vi "Create Input Channels.vi"(8 "error in (no error)":errorcluster, 11 "DAQmx Digitizer in":refnum<class "DAQmx Digitizer.lvclass">) -> (0 "error out":errorcluster, 3 "DAQmx Digitizer out":refnum<class "DAQmx Digitizer.lvclass">)   [LabVIEW 2024, in "DAQmx Digitizer.lvclass"]
uses:
  DAQmx Digitizer.lvclass
  DAQmx Digitizer.lvclass/DAQmx Digitizer.ctl
  Instruments/Pulse Driver/Pulse Driver.lvclass/Pulse Driver.ctl
  Instruments/Instrument Driver/Instrument Driver.lvclass/Instrument Driver.ctl
  Instruments/Pulse Driver/Read Pretrigger samples.vi
  Instruments/Pulse Driver/Read Samples per channel.vi
  Instruments/Instrument Driver/Read Type ID.vi
  Instruments/Pulse Driver/Write t0.vi
  Instruments/Pulse Driver/Write dt.vi
  Instruments/Pulse Driver/Write Set timing from UI.vi
  <vilib>/DAQmx/create/channels.llb/DAQmx Create Channel (AI-Voltage-Basic).vi
  <vilib>/DAQmx/configure/timing.llb/DAQmx Timing (Sample Clock).vi
  <vilib>/DAQmx/configure/trigger.llb/DAQmx Reference Trigger (Digital Edge).vi
  <vilib>/Utility/error.llb/Error Cluster From Error Code.vi
  <vilib>/DAQmx/configure/trigger.llb/DAQmx Start Trigger (Digital Edge).vi
  <vilib>/DAQmx/configure/events/hardwareSignals.llb/DAQmx Export Signal (Most Signals).vi
  <vilib>/ErrorRing/Error Ring.xnode
  <resource>/objmgr/daqmx.rc
  File/File Class/File.lvclass
panel:
  out "CompactDAQ.ChassisDevName":tag
  out "ProductCategory":i32(ring)=14643 items=["M Series DAQ"=14643, "X Series DAQ"=15858, "E Series DAQ"=14642, "S Series DAQ"=14644, "B Series DAQ"=14662, "SC Series DAQ"=14645, "USB DAQ"=14646, "AO Series"=14647, "Digital I/O"=14648, "TIO Series"=14661, "Dynamic Signal Acquisition"=14649, "Switches"=14650, "CompactDAQ Chassis"=14658, "CompactRIO Chassis"=16144, "C Series Module"=14659, "SCXI Module"=14660, "SCC Connector Block"=14704, "SCC Module"=14705, "NI ELVIS"=14755, "Network DAQ"=14829, "SC Express"=15886, "FieldDAQ"=16151, "Unknown"=12588]
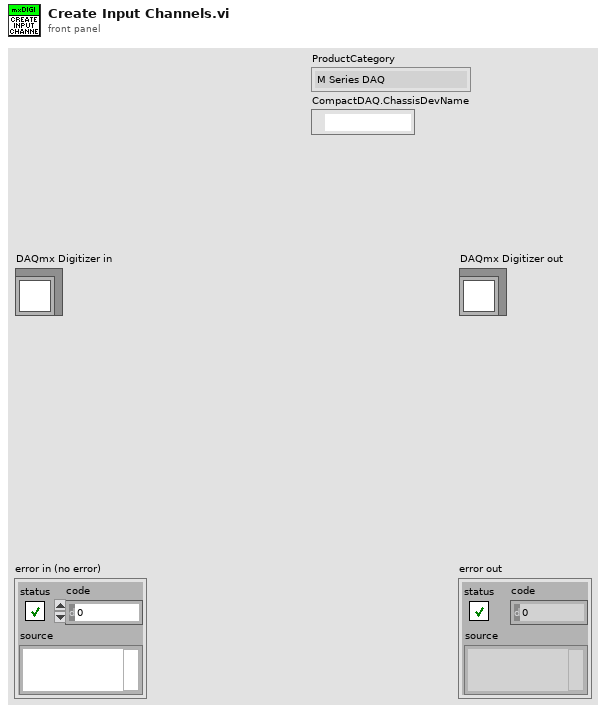
[diagram p1: front panel]
types:
  T1 = typedef "Pusle Driver Configuration.ctl" = cluster{"Post-trigger delay":dbl, "Post-trigger duration":dbl, "Rate":dbl, "Ranges":dbl[], "Re-name channels":string[], "Active channels":string, "External clock":bool}
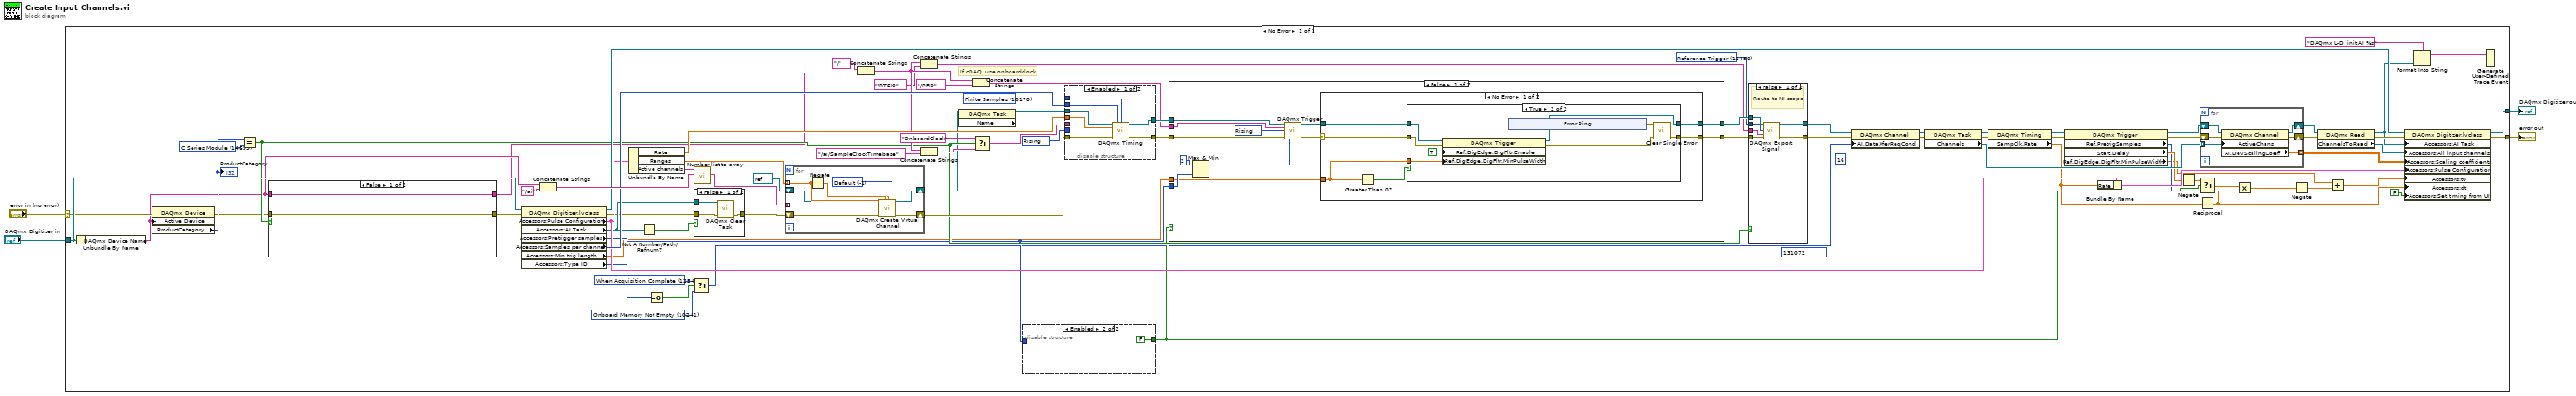
[diagram p0: block diagram]
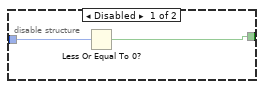
[diagram p3: hidden frame]
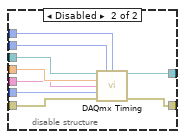
[diagram p4: hidden frame]
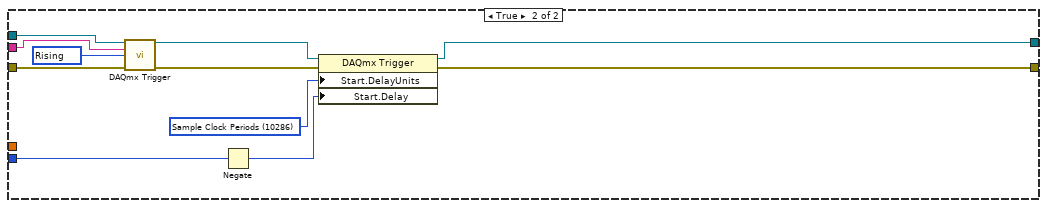
[diagram p7: hidden frame]
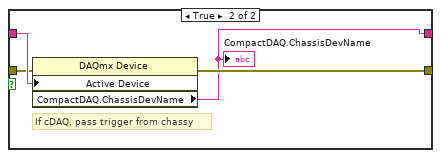
[diagram p8: hidden frame]
diagram:
  n1 = case shown="No Error" "error in (no error)" {
    selector: "error in (no error)" -> [w47 w186]
    tunnel: [w76 w186] -> w3
    tunnel: [w77 w185] -> w1
    tunnel: "DAQmx Digitizer in" -> [w75 w185]
    frame No Error {
      w6 = 10241 items=["Onboard Memory More than Half Full"=10237, "Onboard Memory Not Empty"=10241, "Onboard Memory Custom Threshold"=12577, "When Acquisition Complete"=12546] ("AI.DataXferReqCond")
      w7 = 12546 items=["Onboard Memory More than Half Full"=10237, "Onboard Memory Not Empty"=10241, "Onboard Memory Custom Threshold"=12577, "When Acquisition Complete"=12546] ("AI.DataXferReqCond")
      (unwired) u32 16 ("AI.UsbXferReqCount")
      (unwired) u32 131072 ("AI.UsbXferReqSize")
      w45 = 14659 items=["M Series DAQ"=14643, "X Series DAQ"=15858, "E Series DAQ"=14642, "S Series DAQ"=14644, "B Series DAQ"=14662, "SC Series DAQ"=14645, "USB DAQ"=14646, "AO Series"=14647, "Digital I/O"=14648, "TIO Series"=14661, "Dynamic Signal Acquisition"=14649, "Switches"=14650, "CompactDAQ Chassis"=14658, "CompactRIO Chassis"=16144, "C Series Module"=14659, "SCXI Module"=14660, "SCC Connector Block"=14704, "SCC Module"=14705, "NI ELVIS"=14755, "Network DAQ"=14829, "SC Express"=15886, "FieldDAQ"=16151, "Unknown"=12588] ("ProductCategory")
      w56 = 12490 items=["AI Convert Clock"=12484, "10MHz Reference Clock"=12536, "20MHz Timebase Clock"=12486, "Sample Clock"=12487, "Advance Trigger"=12488, "Reference Trigger"=12490, "Start Trigger"=12491, "Advance Complete Event"=12492, "AI Hold Complete Event"=12493, "Counter Output Event"=12494, "Change Detection Event"=12511, "Watchdog Timer Expired Event"=12512] ("signal")
      w83 = 10280 items=["Rising"=10280, "Falling"=10171] ("active edge")
      w84 = 10178 items=["Finite Samples"=10178, "Continuous Samples"=10123, "Hardware Timed Single Point"=12522] ("sample mode")
      # "If cDAQ, use onboardclock"
      n2 = Unbundle By Name(w75) -> ("DAQmx Device Name"=w39:tag)
      n3 = property class="DAQmx Device"(error in=w47, "Active Device"=w39) -> (error out=w38:errorcluster, "ProductCategory"=w46:i32)  [unwired: 1 in, 1 out]
      "ProductCategory" <- w46
      n4 = Equal?(x=w46, y=w45) -> (x = y?=w40:bool)
      n5 = case shown="False" w40 {
        tunnel: w39 -> [w157 w162]
        tunnel: w38 -> [w158 w161]
        tunnel: [w158 w160] -> w37
        tunnel: [w157 w159] -> w36
        frame False {
        }
        frame True {
          # "If cDAQ, pass trigger from chassy"
          n6 = property class="DAQmx Device"(error in=w161, "Active Device"=w162) -> (error out=w160:errorcluster, "CompactDAQ.ChassisDevName"=w159:tag)  [unwired: 1 in, 1 out]
          "CompactDAQ.ChassisDevName" <- w159
        }
      }
      n7 = property class="DAQmx Digitizer.lvclass"(reference=w75, error in=w37) -> (reference out=w74:refnum<class "DAQmx Digitizer.lvclass">, error out=w24:errorcluster, "Accessors:Pulse Configuration"=w70:T1, "Accessors:AI Task"=w25:refnum<k21>, "Accessors:Pretrigger samples"=w35:i32, "Accessors:Samples per channel"=w71:i32, "Accessors:Min trig length"=w12:dbl, "Accessors:Type ID"=w9:i32)
      n8 = Concatenate Strings(w39, "/ai" ("string")) -> (w80:string)
      n9 = Unbundle By Name(w70) -> ("Rate"=w78:dbl, "Ranges"=w68:dbl[], "Active channels"=w82:string)
      n10 = Not A Number/Path/Refnum?(number/path/refnum=w25) -> (NaN/Path/Refnum?=w26:bool)
      n11 = Equal To 0?(x=w9) -> (x = 0?=w8:bool)
      n12 = Select(t=w7, s=w8, f=w6) -> (s? t:f=w5:i32)
      n13 = call "Number list to array.vi"("Full names prefix"=w80, "Number list"=w82) -> ("Full names"=w79:string[])  [unwired: 6 in, 3 out]
      n14 = case shown="False" w26 {
        tunnel: w25 -> [w91 _]
        tunnel: w24 -> [w90 w92]
        tunnel: [w89 w92] -> w14
        frame False {
          n15 = call <vilib>:"DAQmx Clear Task.vi"("task in"=w91, "error in"=w90) -> ("error out"=w89:errorcluster)  [unwired: 13 in]
        }
        frame True {
        }
      }
      n16 = for {
        tunnel: w79 -> [w184] mode=indexing
        tunnel: w68 -> [w182] mode=indexing
        shift-right: [w179] -> w88
        shift-left: w14 -> [w183]
        shift-right: [w180] -> w16
        shift-left: refnum<k21> refnum ("task out") -> [w177]
        w178 = -1 items=["Default"=-1, "RSE"=10083, "NRSE"=10078, "Differential"=10106, "Pseudodifferential"=12529] ("input terminal configuration")
        n17 = Negate(x=w182) -> (-x=w181:dbl)
        n18 = call-poly <vilib>:"DAQmx Create Virtual Channel.vi"("task in"=w177, "maximum value"=w182, "minimum value"=w181, "input terminal configuration"=w178, "physical channels"=w184, "error in"=w183) -> ("task out"=w180:refnum<k21>, "error out"=w179:errorcluster)  [unwired: 8 in]
      }
      n19 = Concatenate Strings(tag "/" ("string"), w36) -> (w50:string)
      n20 = Concatenate Strings(w50, tag "/RTSI0" ("string")) -> (w51:string)
      n21 = Concatenate Strings(w50, tag "/ai/SampleClockTimebase" ("string")) -> (w44:string)
      n22 = property class="DAQmx Task" props=["Name"](reference=w16) -> (reference out=w15:refnum<k21>)  [unwired: 1 in, 2 out]
      n23 = Concatenate Strings(w50, tag "/PFI0" ("string")) -> (w41:string)
      n24 = Select(t="OnboardClock", s=w40, f=w44) -> (s? t:f=w42:string)
      n25 = disable-structure shown="Enabled" {
        disable-tunnel: w35 -> [w94 _]
        disable-tunnel: [w93 FALSE] -> w33
        frame Disabled {
          n26 = Less Or Equal To 0?(x=w94) -> (x <= 0?=w93:bool)
        }
        frame Enabled {
        }
      }
      n27 = disable-structure shown="Enabled" {
        disable-tunnel: w88 -> [w102 w111]
        disable-tunnel: [w101 w110] -> w87
        disable-tunnel: [w100 w109] -> w86
        disable-tunnel: w84 -> [w99 w108]
        disable-tunnel: w83 -> [_ w107]
        disable-tunnel: w78 -> [w98 w106]
        disable-tunnel: w71 -> [w97 w105]
        disable-tunnel: w15 -> [w96 w104]
        disable-tunnel: w42 -> [_ w103]
        frame Enabled {
          n28 = call-poly <vilib>:"DAQmx Timing.vi"("task/channels in"=w96, "sample mode"=w99, "samples per channel"=w97, "rate"=w98, "error in"=w102) -> ("task out"=w100:refnum<k21>, "error out"=w101:errorcluster)  [unwired: 2 in, 7 out]
        }
        frame Disabled {
          n29 = call-poly <vilib>:"DAQmx Timing.vi"("task/channels in"=w104, "sample mode"=w108, "samples per channel"=w105, "rate"=w106, "source"=w103, "active edge"=w107, "error in"=w111) -> ("task out"=w109:refnum<k21>, "error out"=w110:errorcluster)  [unwired: 7 out]
        }
      }
      n30 = case shown="False" w33 {
        tunnel: w87 -> [w122 w155]
        tunnel: w86 -> [w121 w154]
        tunnel: [w115 w150] -> w57
        tunnel: [w114 w149] -> w55
        tunnel: w41 -> [w120 w153]
        tunnel: w35 -> [w119 w147]
        tunnel: w12 -> [w112 _]
        frame False {
          w123 = 10280 items=["Rising"=10280, "Falling"=10171] ("edge")
          n31 = Max & Min(x=2, y=w119) -> (max(x,y)=w118:i32)  [unwired: 1 out]
          n32 = call-poly <vilib>:"DAQmx Trigger.vi"("task/channels in"=w121, "source"=w120, "edge"=w123, "error in"=w122, "pretrigger samples per channel"=w118) -> ("task out"=w116:refnum<k21>, "error out"=w113:errorcluster)  [unwired: 9 out]
          n33 = case shown="No Error" w113 {
            selector: w113 -> [w126 w145]
            tunnel: w116 -> [w129 w144]
            tunnel: [w128 w144] -> w115
            tunnel: [w127 w145] -> w114
            tunnel: w112 -> [w125 _]
            frame No Error {
              n34 = Greater Than 0?(x=w125) -> (x > 0?=w124:bool)
              n35 = case shown="True" w124 {
                tunnel: w129 -> [w131 w138]
                tunnel: [w131 w137] -> w128
                tunnel: [w130 w135] -> w127
                tunnel: w126 -> [w130 w133]
                tunnel: w125 -> [_ w132]
                frame False {
                }
                frame True {
                  n36 = property class="DAQmx Trigger"(reference=w138, error in=w133, "Ref.DigEdge.DigFltr.Enable"=TRUE, "Ref.DigEdge.DigFltr.MinPulseWidth"=w132) -> (reference out=w137:refnum<k21>, error out=w136:errorcluster)
                  n37 = xnode "Error Ring"() -> ("error out"=w134:errorcluster)
                  n38 = call "Clear Single Error.vi"("Error In"=w136, "Error to clear"=w134) -> ("Error Out"=w135:errorcluster)  [unwired: 8 in, 1 out]
                }
              }
            }
            frame Error {
            }
          }
        }
        frame True {
          w148 = 10286 items=["Sample Clock Periods"=10286, "Seconds"=10364, "Ticks"=10304] ("Start.DelayUnits")
          w156 = 10280 items=["Rising"=10280, "Falling"=10171] ("edge")
          n39 = call-poly <vilib>:"DAQmx Trigger.vi"("task/channels in"=w154, "source"=w153, "edge"=w156, "error in"=w155) -> ("task out"=w152:refnum<k21>, "error out"=w151:errorcluster)  [unwired: 10 out]
          n40 = Negate(x=w147) -> (-x=w146:i32)
          n41 = property class="DAQmx Trigger"(reference=w152, error in=w151, "Start.DelayUnits"=w148, "Start.Delay"=w146) -> (reference out=w150:refnum<k21>, error out=w149:errorcluster)
        }
      }
      n42 = case shown="False" w40 {
        tunnel: w57 -> [w168 w170]
        tunnel: w56 -> [w167 _]
        tunnel: w55 -> [w166 w169]
        tunnel: [w165 w169] -> w54
        tunnel: w51 -> [w164 _]
        tunnel: [w163 w170] -> w48
        frame False {
          # "Route to NI scope"
          n43 = call-poly <vilib>:"DAQmx Export Signal.vi"("task/channels in"=w168, "signal"=w167, "output terminal"=w164, "error in"=w166) -> ("task out"=w163:refnum<k21>, "error out"=w165:errorcluster)  [unwired: 10 in]
        }
        frame True {
          # "ignore for\ncDAQ"
        }
      }
      n44 = property class="DAQmx Channel"(reference=w48, error in=w54, "AI.DataXferReqCond"=w5) -> (reference out=w29:refnum<k21>, error out=w28:errorcluster)
      n45 = property class="DAQmx Task"(reference=w29, error in=w28) -> (reference out=w73:refnum<k21>, error out=w72:errorcluster, "Channels"=w67:refnum<k21>[])
      n46 = property class="DAQmx Timing"(reference=w73, error in=w72) -> (reference out=w65:refnum<k21>, error out=w62:errorcluster, "SampClk.Rate"=w66:dbl)
      n47 = property class="DAQmx Trigger"(reference=w65, error in=w62) -> (reference out=w64:refnum<k21>, error out=w63:errorcluster, "Ref.PretrigSamples"=w31:u32, "Start.Delay"=w34:dbl, "Ref.DigEdge.DigFltr.MinPulseWidth"=w10:dbl)
      n48 = Bundle By Name(cluster=w70, "Rate"=w66) -> (w69:T1)
      n49 = Negate(x=w34) -> (-x=w32:dbl)
      n50 = Select(t=w32, s=w33, f=w31) -> (s? t:f=w30:dbl)
      n51 = Reciprocal(x=w66) -> (1/x=w61:dbl)
      n52 = for {
        tunnel: w67 -> [w176] mode=indexing
        shift-right: [w173] -> w23
        shift-left: w64 -> [w174]
        shift-right: [w172] -> w21
        shift-left: w63 -> [w175]
        tunnel: [w171] -> w27 mode=indexing
        n53 = property class="DAQmx Channel"(reference=w174, error in=w175, "ActiveChans"=w176) -> (reference out=w173:refnum<k21>, error out=w172:errorcluster, "AI.DevScalingCoeff"=w171:dbl[])
      }
      n54 = Multiply(x=w30, y=w61) -> (x*y=w60:dbl)
      n55 = Negate(x=w60) -> (-x=w58:dbl)
      n56 = property class="DAQmx Read"(reference=w23, error in=w21) -> (reference out=w17:refnum<k21>, error out=w20:errorcluster, "ChannelsToRead"=w22:refnum<k21>)
      n57 = Add(x=w10, y=w58) -> (x+y=w11:dbl)
      n58 = property class="DAQmx Digitizer.lvclass"(reference=w74, error in=w20, "Accessors:AI Task"=w17, "Accessors:All input channels"=w22, "Accessors:Scaling coefficients"=w27, "Accessors:Pulse Configuration"=w69, "Accessors:t0"=w11, "Accessors:dt"=w61, "Accessors:Set timing from UI"=FALSE ("Set timing from UI")) -> (reference out=w77:refnum<class "DAQmx Digitizer.lvclass">, error out=w76:errorcluster)
      n59 = Format Into String(format string="DAQmx L-D  init AI %s" ("string"), w17) -> (resulting string=w18:string)  [unwired: 2 in, 1 out]
      n60 = Generate User-Defined Trace Event(2:w18) -> ()  [unwired: 1 in]
    }
    frame Error {
    }
  }
  "error out" <- w3
  "DAQmx Digitizer out" <- w1
